vi "二进制转化.vi"(11 "一致性结果字符串":string="0010100000000000") -> (3 "字符串":string)   [LabVIEW 2017]
panel:
  out "数字":i32 format="%04d"
  out "子字符串":string
  # "2"
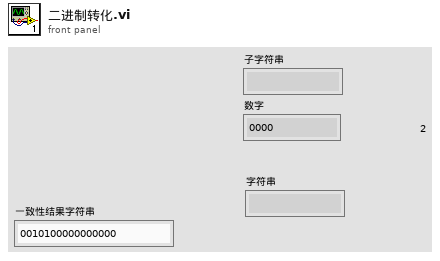
[diagram p1: front panel]
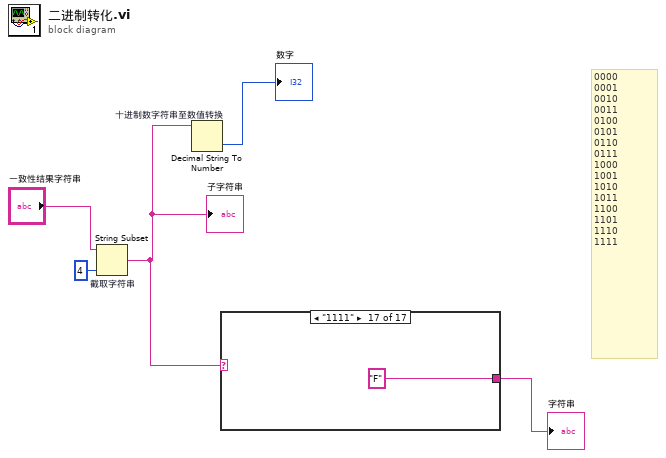
[diagram p0: block diagram]
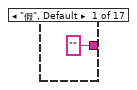
[diagram p2: hidden frame]
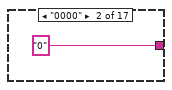
[diagram p3: hidden frame]
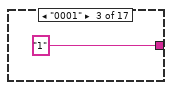
[diagram p4: hidden frame]
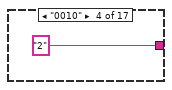
[diagram p5: hidden frame]
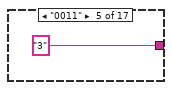
[diagram p6: hidden frame]
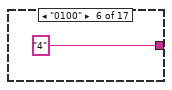
[diagram p7: hidden frame]
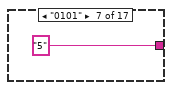
[diagram p8: hidden frame]
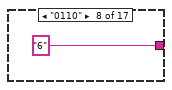
[diagram p9: hidden frame]
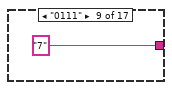
[diagram p10: hidden frame]
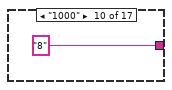
[diagram p11: hidden frame]
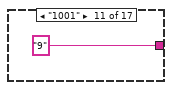
[diagram p12: hidden frame]
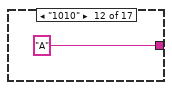
[diagram p13: hidden frame]
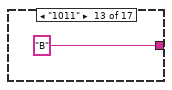
[diagram p14: hidden frame]
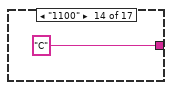
[diagram p15: hidden frame]
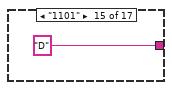
[diagram p16: hidden frame]
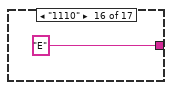
[diagram p17: hidden frame]
diagram:
  # "0000\n0001\n0010\n0011\n0100\n0101\n0110\n0111\n1000\n1001\n1010\n1011\n1100\n1101\n1110\n1111"
  n1 = String Subset "截取字符串"(string="一致性结果字符串", length (rest)=4 ("长度（剩余）")) -> (substring=w2:string)  [unwired: 1 in]
  "子字符串" <- w2
  n2 = Decimal String To Number "十进制数字符串至数值转换"(string=w2) -> (number=→"数字":i32)  [unwired: 2 in, 1 out]
  n3 = case shown="\"1111\"" w2 {
    tunnel: ["" "0" "1" "2" "3" "4" "5" "6" "7" "8" "9" "A" "B" "C" "D" "E" "F"] -> w1
    frame "假", Default {
    }
    frame "0000" {
    }
    frame "0001" {
    }
    frame "0010" {
    }
    frame "0011" {
    }
    frame "0100" {
    }
    frame "0101" {
    }
    frame "0110" {
    }
    frame "0111" {
    }
    frame "1000" {
    }
    frame "1001" {
    }
    frame "1010" {
    }
    frame "1011" {
    }
    frame "1100" {
    }
    frame "1101" {
    }
    frame "1110" {
    }
    frame "1111" {
    }
  }
  "字符串" <- w1
